vi "LaserMaster.vi"() -> ()   [LabVIEW 2010]
uses:
  <vilib>/Instr/_visa.llb/VISA Configure Serial Port (Instr).vi
  <vilib>/Utility/file.llb/Write To Spreadsheet File (string).vi
panel:
  out "Start time":timestamp
  out "Step":dbl
  out "State next step":string
  in  "stop":bool
  out "Query backup List":string[][](array[string])=[["?L", " 0\r"], ["?K", " 0\r"], ["?F", " 0\r"], ["?FH", " 2\r"], ["?SHUTTER", " 0\r"], ["?UF", " 0\r"], ["?PHLDC", " 1\r"], ["?PZTMC", " 0\r"], ["?PZTXC", " 2.24\r"], ["?PZTYC", " 2.14\r"], ["?PHLDP", " 0\r"], ["?PZTMP", " 0\r"], ["?PZTXP", " 2.58\r"], ["?PXTYP", "  Query Error:?PXTYP\r"], ["?PTRK", "  Query Error:?PTRK\r"], ["?MDLK", " 0\r"], ["?PP", " 0.80\r"], ["?TS", " 0\r"], ["?SM", " 1\r"], ["?HM", " 1\r"], ["?VW", " 850\r"], ["?STPRPOS", " 2096\r"], ["?C", " 0.00\r"], ["?D1C", " 0.08\r"], ["?D2C", " -0.43\r"], ["?BT", " 20.07\r"], ["?D1T", " 24.20\r"], ["?D2T", " 24.20\r"], ["?VT", " 20.72\r"], ["?LBOT", " 148.45\r"], ["?ET", " 39.01\r"], ["?D1ST", " 24.20\r"], ["?D2ST", " 24.20\r"], ["?VST", " 30.00\r"], ["?LBOST", " 148.41\r"], ["?EST", " 39.00\r"], ["?D1TD", " 500.12\r"], ["?D2TD", " 464.53\r"], ["?VD", " 0.00\r"], ["?LBOD", " 5358.08\r"], ["?ED", " 2152.46\r"], ["?D1HST", " 21.35\r"], ["?D2HST", " 21.48\r"], ["?LBOH", " 1\r"], ["?LRS", " 2\r"], ["?D1SS", " 1\r"], ["?D2SS", " 1\r"], ["?VSS", " 0\r"], ["?LBOSS", " 1\r"], ["?ESS", " 1\r"], ["?D1H", "  351.54\r"], ["?D2H", "  351.52\r"], ["?HH", " 37\r"], ["?D1V", " 0.19\r"], ["?D2V", " 0.18\r"], ["?SV", " 8.26,8.26,9.57\r"], ["?MB", "  Query Error:?MB\r"], ["?PI", " 2BC\r"], ["?BV", " 13.24\r"], ["?AMDLK", " 1\r"], ["?PZTS", "  Query Error:?PZTS\r"], ["?TMAX", " 1080\r"], ["?TMIN", " 680\r"], ["?ALIGN", " 0\r"], ["?ALIGNP", " 250\r"], ["?ALIGNW", " 730\r"], ["?LFP", " 0\r"], ["?PZTXCM", " 8.11\r"], ["?PZTXCP", " -10.30\r"], ["?PZTXPM", " 8.11\r"], ["?PZTXPP", " 3.06\r"], ["?PZTYCM", " 8.11\r"], ["?PZTYCP", " -14.28\r"], ["?PZTYPM", " 8.11\r"], ["?PZTYPP", " 11.74\r"], ["?RH", " 0\r"], ["?SN", " 9571\r"], ["?ST", " Standby\r"], ["?GDDCURVE", " 0\r"], ["?GDD", " 0\r"], ["?GDDCURVEN", " ZERO\r"], ["?CURVEN", " OUT OF RANGE\r"], ["?COMP", " 1\r"], ["?HMCOMP", " 1\r"], ["?GDDMAX", " 17333\r"], ["?GDDMIN", "0"]]
  out "Laser Info":i32
  out "Shutter off time":dbl
  out "Quiting":dbl
  out "Backuper state":string
  in  "Tab Control":T1(tab)
  out "Laser Status":bool
  out "Power (mW)":dbl(knob) scale=0.0..5000.0
  out "Walking":bool
  out "Sleeping":bool
  out "ModeLocked":bool
  out "Backing up":bool
  in  "Dither hold":bool
  in  "Shutter":bool
  in  "Wavelength":dbl
  in  "GDD":dbl
  in  "Align":bool
  in  "QUIT":bool
  out "Max":string
  in  "Home motor":bool
  in  "Optimize":bool
  in  "WV Walk":bool
  in  "Auto-Standby\nTime (min)":dbl=120.0
  in  "Sleep":bool
  in  "Backup":bool
  in  "Auto-Backup \nIdle Time (min)":dbl=30.0
  out "Operating Status":string
  out "Tunning Status":i32
  out "Idle Time":dbl format="%.1f"
  out "Laser On Time":dbl format="%#.1f"
  in  "Laser Control":bool
  in  "Refresh":bool
  out "Query List":string[][](array[string])
  out "queue #":i32
  in  "Command Line":string
  out "Laser Response":string
  # "LASER"
  # "LASER fine-tune"
  # "BACKUP"
  # "Timers"
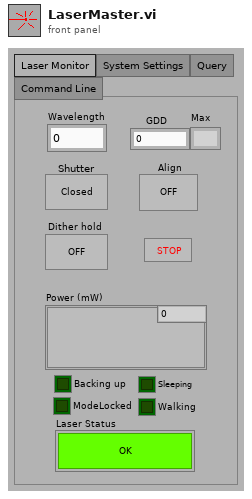
[diagram p1: front panel]
types:
  T1 = enum32{"Laser Monitor", "System Settings", "Query", "Command Line"}
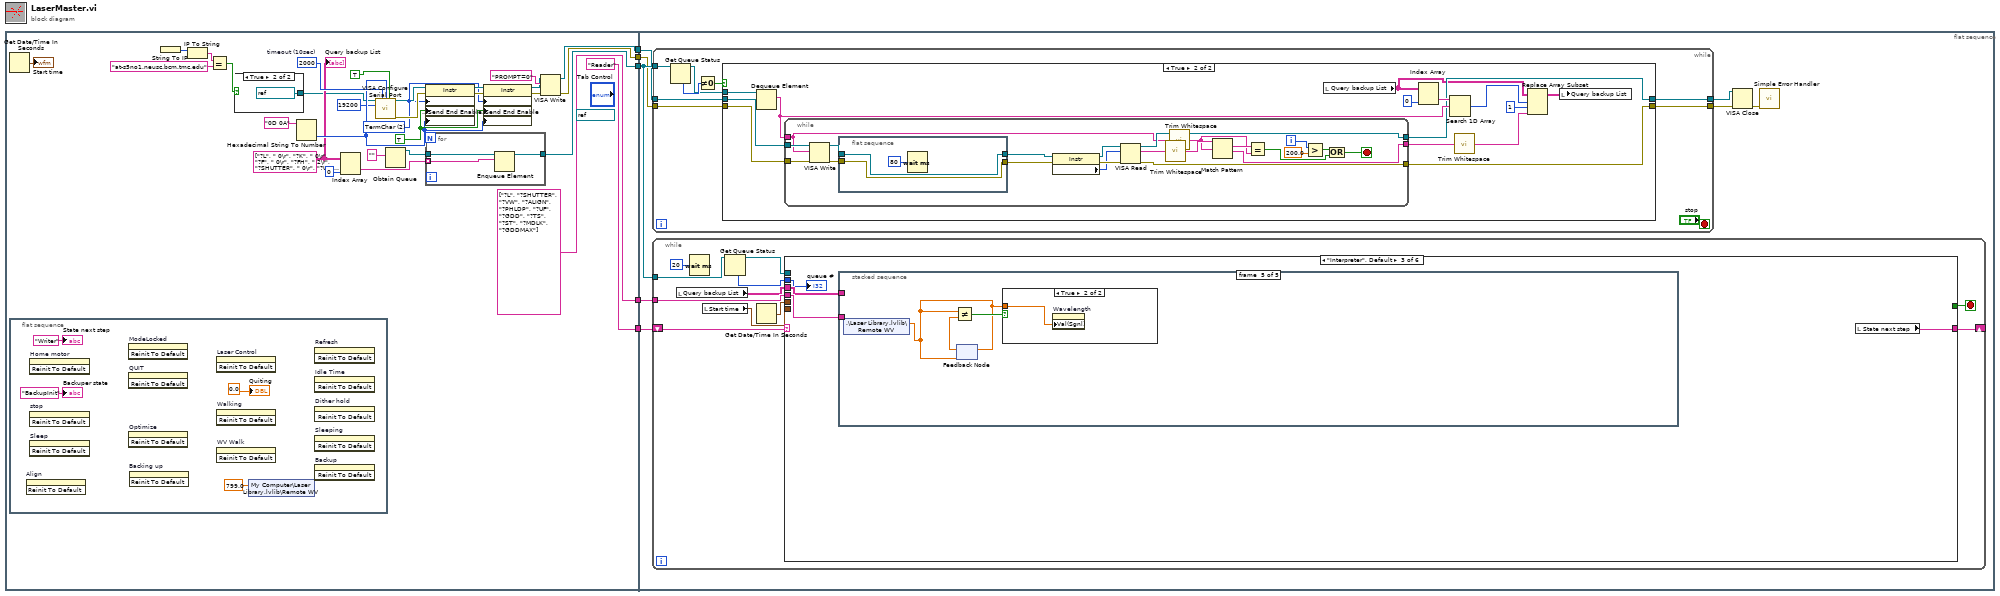
[diagram p0: block diagram]
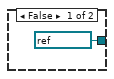
[diagram p2: hidden frame]
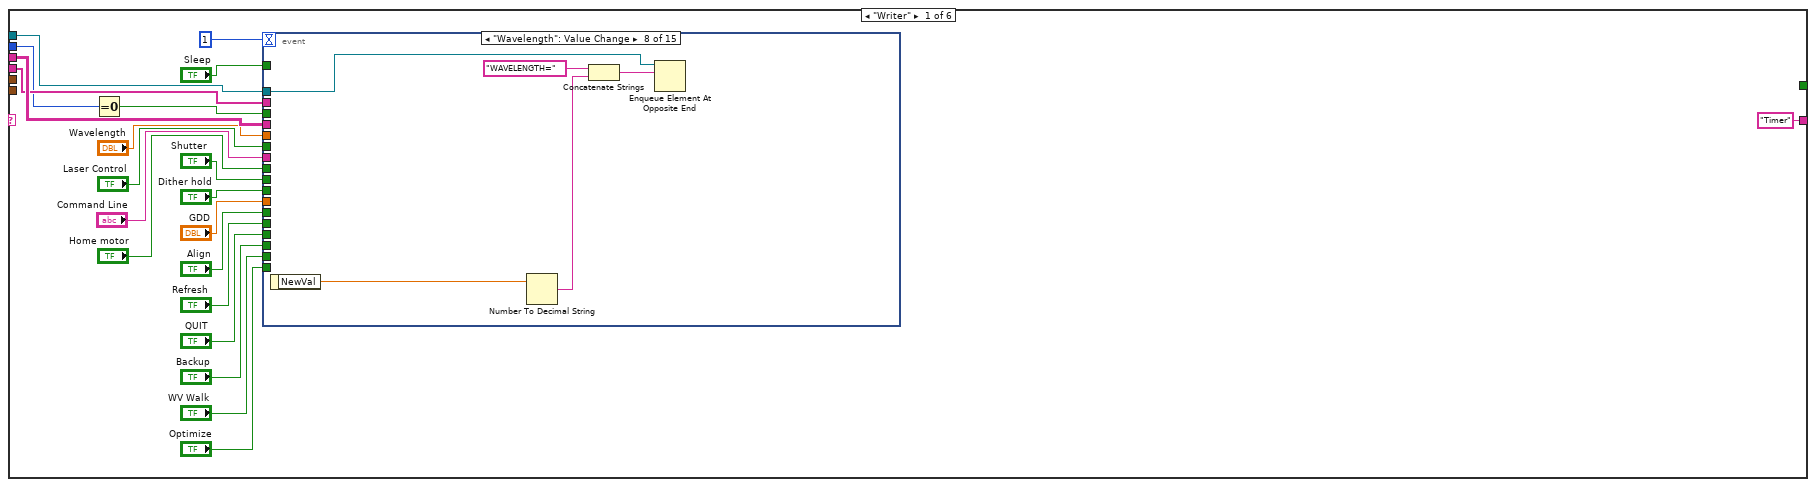
[diagram p4: hidden frame]
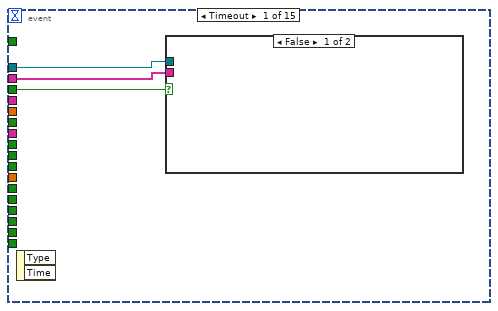
[diagram p5: hidden frame]
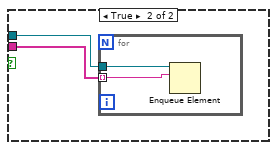
[diagram p6: hidden frame]
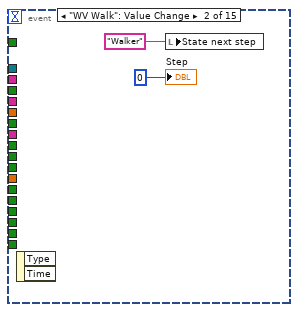
[diagram p7: hidden frame]
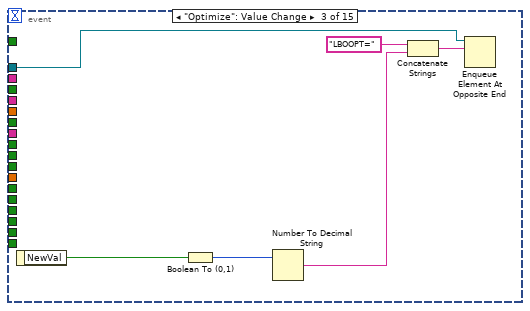
[diagram p8: hidden frame]
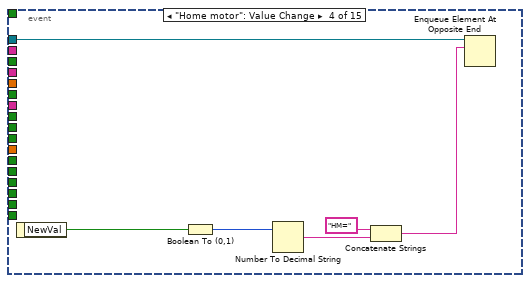
[diagram p9: hidden frame]
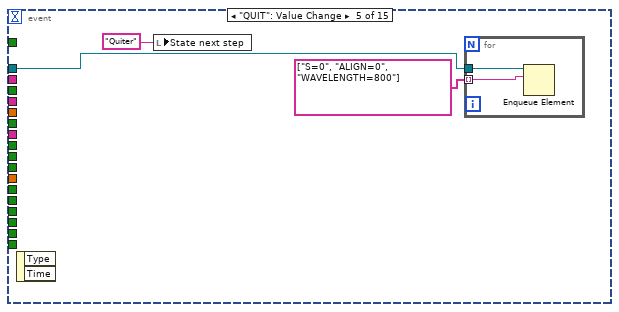
[diagram p10: hidden frame]
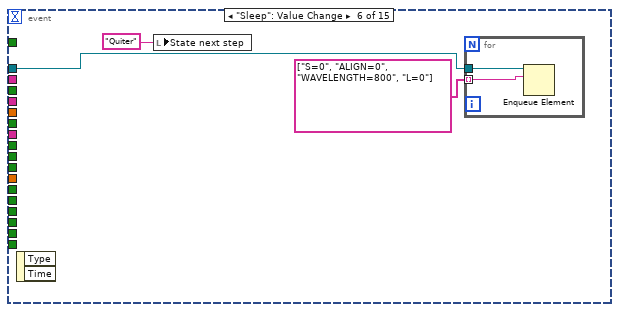
[diagram p11: hidden frame]
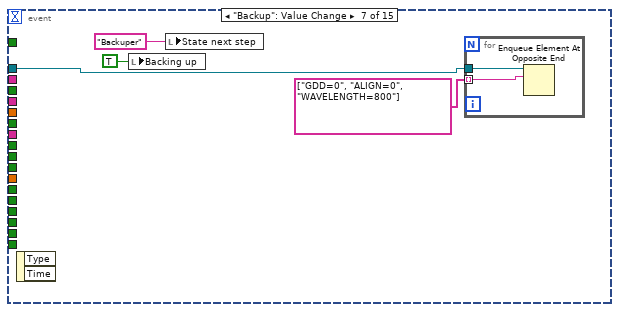
[diagram p12: hidden frame]
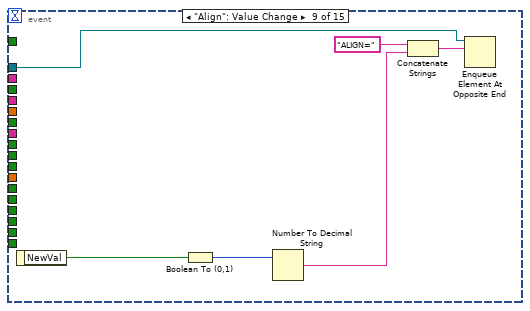
[diagram p13: hidden frame]
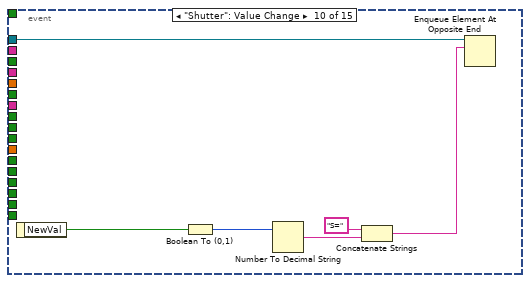
[diagram p14: hidden frame]
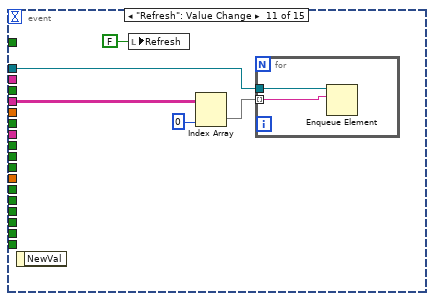
[diagram p15: hidden frame]
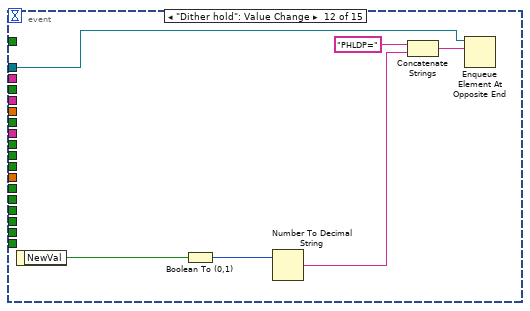
[diagram p16: hidden frame]
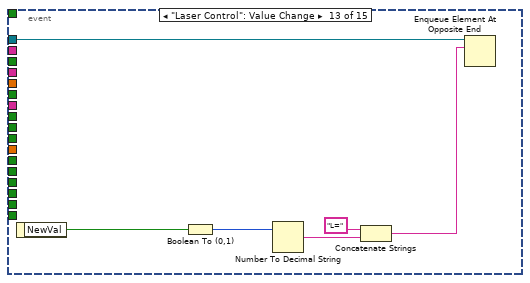
[diagram p17: hidden frame]
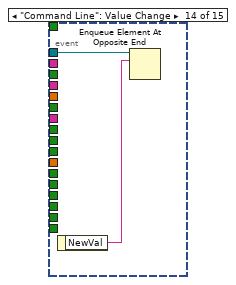
[diagram p18: hidden frame]
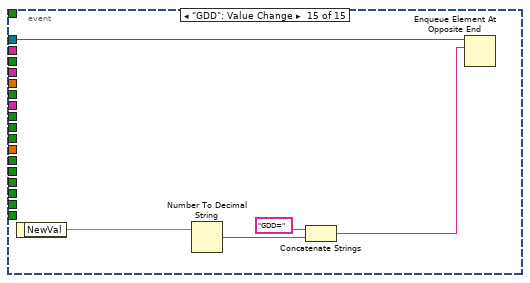
[diagram p19: hidden frame]
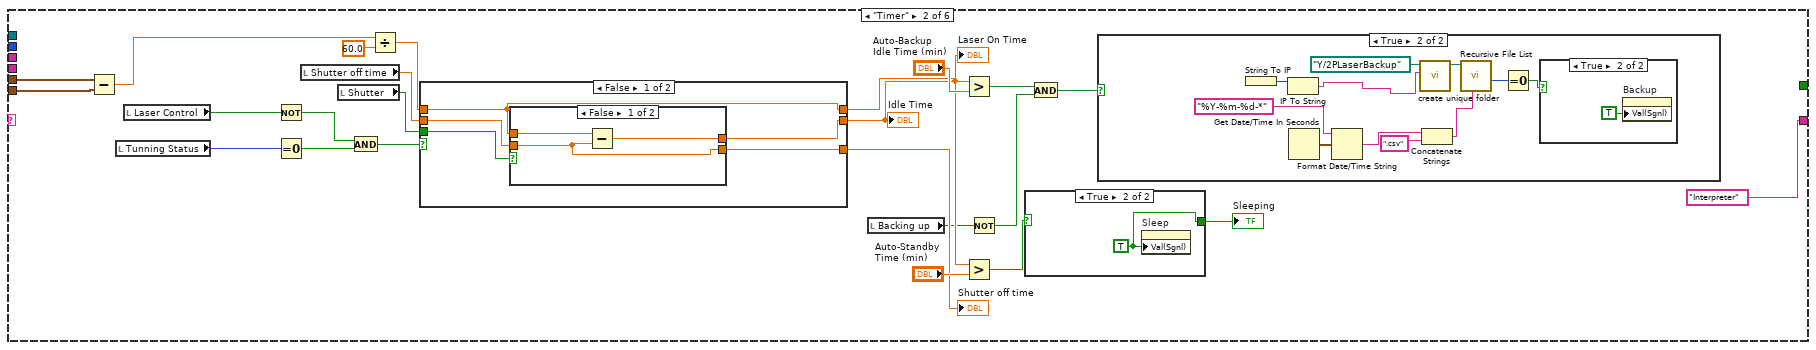
[diagram p20: hidden frame]
diagram:
  n1 = flat-sequence {
    tunnel: [w24] -> w5
    tunnel: [w23] -> w4
    tunnel: [w14] -> w3
    tunnel: [string[] ["?L", "?SHUTTER", "?VW", "?ALIGN", "?PHLDP", "?UF", "?GDD", "?TS", "?ST", "?MDLK", "?GDDMAX"]] -> w2
    tunnel: ["Reader"] -> w1
    tunnel: w5 -> [w48]
    tunnel: w4 -> [w45]
    tunnel: w3 -> [w49]
    tunnel: w2 -> [w51]
    tunnel: w1 -> [w50]
    frame #0 {
      (unwired) refnum<visa-resource-name> "COM1" ("VISA resource name")
      w13 = string[][] [["?L", " 0\r"], ["?K", " 0\r"], ["?F", " 0\r"], ["?FH", " 2\r"], ["?SHUTTER", " 0\r"], ["?UF", " 0\r"], ["?PHLDC", " 1\r"], ["?PZTMC", " 0\r"], ["?PZTXC", " 2.24\r"], ["?PZTYC", " 2.14\r"], ["?PHLDP", " 0\r"], ["?PZTMP", " 0\r"], ["?PZTXP", " 2.58\r"], ["?PXTYP", "  Query Error:?PXTYP\r"], ["?PTRK", "  Query Error:?PTRK\r"], ["?MDLK", " 0\r"], ["?PP", " 0.80\r"], ["?TS", " 0\r"], ["?SM", " 1\r"], ["?HM", " 1\r"], ["?VW", " 850\r"], ["?STPRPOS", " 2096\r"], ["?C", " 0.00\r"], ["?D1C", " 0.08\r"], ["?D2C", " -0.43\r"], ["?BT", " 20.07\r"], ["?D1T", " 24.20\r"], ["?D2T", " 24.20\r"], ["?VT", " 20.72\r"], ["?LBOT", " 148.45\r"], ["?ET", " 39.01\r"], ["?D1ST", " 24.20\r"], ["?D2ST", " 24.20\r"], ["?VST", " 30.00\r"], ["?LBOST", " 148.41\r"], ["?EST", " 39.00\r"], ["?D1TD", " 500.12\r"], ["?D2TD", " 464.53\r"], ["?VD", " 0.00\r"], ["?LBOD", " 5358.08\r"], ["?ED", " 2152.46\r"], ["?D1HST", " 21.35\r"], ["?D2HST", " 21.48\r"], ["?LBOH", " 1\r"], ["?LRS", " 2\r"], ["?D1SS", " 1\r"], ["?D2SS", " 1\r"], ["?VSS", " 0\r"], ["?LBOSS", " 1\r"], ["?ESS", " 1\r"], ["?D1H", "  351.54\r"], ["?D2H", "  351.52\r"], ["?HH", " 37\r"], ["?D1V", " 0.19\r"], ["?D2V", " 0.18\r"], ["?SV", " 8.26,8.26,9.57\r"], ["?MB", "  Query Error:?MB\r"], ["?PI", " 2BC\r"], ["?BV", " 13.24\r"], ["?AMDLK", " 1\r"], ["?PZTS", "  Query Error:?PZTS\r"], ["?TMAX", " 1080\r"], ["?TMIN", " 680\r"], ["?ALIGN", " 0\r"], ["?ALIGNP", " 250\r"], ["?ALIGNW", " 730\r"], ["?LFP", " 0\r"], ["?PZTXCM", " 8.11\r"], ["?PZTXCP", " -10.30\r"], ["?PZTXPM", " 8.11\r"], ["?PZTXPP", " 3.06\r"], ["?PZTYCM", " 8.11\r"], ["?PZTYCP", " -14.28\r"], ["?PZTYPM", " 8.11\r"], ["?PZTYPP", " 11.74\r"], ["?RH", " 0\r"], ["?SN", " 9571\r"], ["?ST", " Standby\r"], ["?GDDCURVE", " 0\r"], ["?GDD", " 0\r"], ["?GDDCURVEN", " ZERO\r"], ["?CURVEN", " OUT OF RANGE\r"], ["?COMP", " 1\r"], ["?HMCOMP", " 1\r"], ["?GDDMAX", " 17333\r"], ["?GDDMIN", "0"]] ("Query backup List")
      w27 = TRUE ("Message Based Settings:Send End Enable")
      w28 = u16 2 items=["None", "LastBit", "TermChar", "Break"] ("Serial Settings:Serial End Mode for Writes")
      w35 = u32 2000  # timeout (10sec)
      n2 = Get Date/Time In Seconds() -> (seconds since 1Jan1904=→"Start time":timestamp)
      n3 = flat-sequence {
        frame #0 {
          n4 = invoke on="Align" class="Bool (strict)" method="Reinit To Default"() -> ()  [unwired: 3 in, 3 out]
          n5 = invoke on="Home motor" class="Bool" method="Reinit To Default"() -> ()  [unwired: 3 in, 3 out]
          n6 = invoke on="stop" class="Bool (strict)" method="Reinit To Default"() -> ()  [unwired: 3 in, 3 out]
          n7 = invoke on="Sleep" class="Bool (strict)" method="Reinit To Default"() -> ()  [unwired: 3 in, 3 out]
          n8 = invoke on="ModeLocked" class="Bool (strict)" method="Reinit To Default"() -> ()  [unwired: 3 in, 3 out]
          n9 = invoke on="QUIT" class="Bool (strict)" method="Reinit To Default"() -> ()  [unwired: 3 in, 3 out]
          n10 = invoke on="Optimize" class="Bool" method="Reinit To Default"() -> ()  [unwired: 3 in, 3 out]
          n11 = invoke on="Backing up" class="Bool (strict)" method="Reinit To Default"() -> ()  [unwired: 3 in, 3 out]
          n12 = invoke on="Laser Control" class="Bool (strict)" method="Reinit To Default"() -> ()  [unwired: 3 in, 3 out]
          n13 = invoke on="Walking" class="Bool (strict)" method="Reinit To Default"() -> ()  [unwired: 3 in, 3 out]
          n14 = invoke on="WV Walk" class="Bool (strict)" method="Reinit To Default"() -> ()  [unwired: 3 in, 3 out]
          n15 = shared-variable "My Computer\\Laser Library.lvlib\\Remote WV"(799.0 ("Remote WV")) -> ()  [unwired: 1 in, 1 out]
          n16 = invoke on="Refresh" class="Bool (strict)" method="Reinit To Default"() -> ()  [unwired: 3 in, 3 out]
          n17 = invoke on="Idle Time" class="DigNum (strict)" method="Reinit To Default"() -> ()  [unwired: 3 in, 3 out]
          n18 = invoke on="Dither hold" class="Bool (strict)" method="Reinit To Default"() -> ()  [unwired: 3 in, 3 out]
          n19 = invoke on="Sleeping" class="Bool (strict)" method="Reinit To Default"() -> ()  [unwired: 3 in, 3 out]
          n20 = invoke on="Backup" class="Bool (strict)" method="Reinit To Default"() -> ()  [unwired: 3 in, 3 out]
          "Backuper state" <- "BackupInit"
          "Quiting" <- 0.0 ("Quiting")
          "State next step" <- "Writer"
        }
      }
      n21 = String To IP() -> (0:w10:u32)  [unwired: 1 in]
      n22 = IP To String(2:w10) -> (0:w9:string)  [unwired: 1 in]
      n23 = Equal?(x=w9, y="at-s5no1.neusc.bcm.tmc.edu") -> (x = y?=w6:bool)
      n24 = case shown="True" w6 {
        tunnel: [refnum<visa-resource-name> "COM1" ("VISA resource name") refnum<visa-resource-name> "COM5" ("VISA resource name")] -> w7
        frame False {
        }
        frame True {
        }
      }
      n25 = Hexadecimal String To Number(string="0D 0A") -> (number=w26:u32)  [unwired: 2 in, 1 out]
      n26 = Index Array(array=w13, index (col)=0 ("disabled index (col)")) -> (element=w16:string[])  [unwired: 1 in]
      n27 = call-poly "VISA Configure Serial Port"("VISA resource name"=w7, "timeout (10sec)"=w35, "termination char\n(0xA = '\\n' = LF)"=w26, "Enable Termination\nChar (T)"=TRUE ("Enable Termination\nChar (T)"), "baud rate (9600)"=u32 19200) -> ("VISA resource name out"=w32:refnum<visa-resource-name>, "error out"=w31:errorcluster)  [unwired: 5 in, 4 out]
      n28 = Obtain Queue(element data type="") -> (queue out=w18:refnum<queue>)  [unwired: 4 in, 2 out]
      n29 = property class="Instr"(reference=w32, error in=w31, "Serial Settings:End Mode for Writes"=w28, "Message Based Settings:Send End Enable"=w27, "Message Based Settings:Termination Character"=w26) -> (reference out=w30:refnum<visa-resource-name>, error out=w29:errorcluster)
      n30 = for {
        tunnel: w18 -> [w44]
        tunnel: w16 -> [w43] mode=indexing
        tunnel: [w42] -> w14
        n31 = Enqueue Element(queue=w44, element=w43) -> (queue out=w42:refnum<queue>)  [unwired: 2 in, 2 out]
      }
      n32 = property class="Instr"(reference=w30, error in=w29, "Serial Settings:End Mode for Writes"=w28, "Message Based Settings:Send End Enable"=w27, "Message Based Settings:Termination Character"=w26) -> (reference out=w21:refnum<visa-resource-name>, error out=w20:errorcluster)
      n33 = VISA Write(VISA resource name=w21, write buffer="PROMPT=0", error in (no error)=w20) -> (VISA resource name out=w24:refnum<visa-resource-name>, error out=w23:errorcluster)  [unwired: 1 out]
      "Query backup List" <- w13
    }
    frame #1 {
      n34 = while {
        tunnel: w49 -> [w56]
        tunnel: w48 -> [w61]
        tunnel: [w60] -> w47
        tunnel: [w59] -> w46
        tunnel: w45 -> [w58]
        stop <- "stop" stop-if-true
        n35 = Get Queue Status(queue=w56) -> (queue out=w53:refnum<queue>, # elements in queue=w55:i32)  [unwired: 2 in, 6 out]
        n36 = Not Equal To 0?(x=w55) -> (x != 0?=w54:bool)
        n37 = case shown="True" w54 {
          tunnel: w53 -> [_ w70]
          tunnel: w61 -> [w63 w69]
          tunnel: [w63 w68] -> w60
          tunnel: [w62 w67] -> w59
          tunnel: w58 -> [w62 w66]
          frame False {
          }
          frame True {
            n38 = Dequeue Element(queue=w70) -> (element=w72:string)  [unwired: 2 in, 3 out]
            n39 = while {
              tunnel: w69 -> [w99]
              tunnel: w66 -> [w98]
              tunnel: [w97] -> w68
              tunnel: [w96] -> w67
              tunnel: w72 -> [w84]
              tunnel: [w92] -> w73
              i -> [w82]
              stop <- w79 stop-if-true
              n40 = VISA Write(VISA resource name=w99, write buffer=w84, error in (no error)=w98) -> (VISA resource name out=w90:refnum<visa-resource-name>, error out=w87:errorcluster)  [unwired: 1 out]
              n41 = flat-sequence {
                tunnel: [w102] -> w89
                tunnel: w90 -> [w102]
                tunnel: w87 -> [w101]
                tunnel: [w101] -> w88
                frame #0 {
                  n42 = Wait (ms)(milliseconds to wait=u32 80) -> ()  [unwired: 1 out]
                }
              }
              n43 = property class="Instr"(reference=w89, error in=w88) -> (reference out=w95:refnum<visa-resource-name>, error out=w94:errorcluster, "Serial Settings:Number of Bytes at Serial Port"=w93:u32)
              n44 = VISA Read(VISA resource name=w95, byte count=w93, error in (no error)=w94) -> (VISA resource name out=w97:refnum<visa-resource-name>, read buffer=w86:string, error out=w96:errorcluster)  [unwired: 1 out]
              n45 = call <vilib>:"Trim Whitespace.vi"("string"=w86) -> ("trimmed string"=w85:string)  [unwired: 1 in]
              n46 = call <vilib>:"Trim Whitespace.vi"("string"=w84) -> ("trimmed string"=w78:string)  [unwired: 1 in]
              n47 = Match Pattern(string=w85, regular expression=w78) -> (match substring=w91:string, after substring=w92:string)  [unwired: 1 in, 2 out]
              n48 = Equal?(x=w91, y=w78) -> (x = y?=w80:bool)
              n49 = Greater?(x=w82, y=200.0) -> (0:w81:bool)
              n50 = Compound Arithmetic op=OR(w81, w80) -> (w79:bool)
            }
            n51 = local read "Query backup List"() -> (w65:string[][])
            n52 = Index Array(array=w65, index (col)=0 ("index (row)")) -> (element=w76:string[])  [unwired: 1 in]
            n53 = Search 1D Array(1D array=w76, element=w72) -> (index of element=w74:i32)  [unwired: 1 in]
            n54 = call <vilib>:"Trim Whitespace.vi"("string"=w73) -> ("trimmed string"=w71:string)  [unwired: 1 in]
            n55 = Replace Array Subset(array=w65, new element=w71, index (row)=w74, index (col)=1 ("disabled index (col)")) -> (w64:string[][])
            n56 = local write "Query backup List"(w64) -> ()
          }
        }
      }
      n57 = while {
        tunnel: w49 -> [w110]
        tunnel: w51 -> [w111]
        shift-right: [w112] -> _
        shift-left: w50 -> [w113]
        stop <- w107 stop-if-true
        n58 = local read "Query backup List"() -> (w109:string[][])
        n59 = Wait (ms)(milliseconds to wait=u32 20) -> ()  [unwired: 1 out]
        n60 = local read "Start time"() -> (w103:timestamp)
        n61 = Get Queue Status(queue=w110) -> (queue out=w106:refnum<queue>, # elements in queue=w105:i32)  [unwired: 2 in, 6 out]
        n62 = Get Date/Time In Seconds() -> (seconds since 1Jan1904=w104:timestamp)
        n63 = case shown="\"Interpreter\", Default" w113 {
          tunnel: w106 -> [w134 _ _ _ _ _]
          tunnel: w109 -> [w133 _ w267 _ w400 _]
          tunnel: w111 -> [w132 _ w268 _ _ _]
          tunnel: ["Timer" "Interpreter" w266 "Writer" "Writer" w425] -> w112
          tunnel: w105 -> [w131 _ w265 _ _ w427]
          tunnel: [_ _ _ _ _ w424] -> w107
          tunnel: w104 -> [_ w218 _ _ _ _]
          tunnel: w103 -> [_ w216 _ _ _ _]
          frame "Writer" {
            n64 = Equal To 0?(x=w131) -> (x = 0?=w119:bool)
            n65 = event shown="[7] \"Wavelength\": Value Change" {
              selector: _ -> [_ _ _ _ _ _ _ _ _ _ _ _ _ _ _]
              dyn-events: _ -> [_ _ _ _ _ _ _ _ _ _ _ _ _ _ _]
              timeout: 1 -> [_ _ _ _ _ _ _ _ _ _ _ _ _ _ _]
              tunnel: w134 -> [w137 _ w144 w151 w157 w161 w168 w173 w178 w184 w190 w197 w202 w209 w211]
              tunnel: "Shutter" -> [_ _ _ _ _ _ _ _ _ _ _ _ _ _ _]
              tunnel: "Dither hold" -> [_ _ _ _ _ _ _ _ _ _ _ _ _ _ _]
              tunnel: "GDD" -> [_ _ _ _ _ _ _ _ _ _ _ _ _ _ _]
              tunnel: "Align" -> [_ _ _ _ _ _ _ _ _ _ _ _ _ _ _]
              tunnel: "Wavelength" -> [_ _ _ _ _ _ _ _ _ _ _ _ _ _ _]
              tunnel: "Laser Control" -> [_ _ _ _ _ _ _ _ _ _ _ _ _ _ _]
              tunnel: "Command Line" -> [_ _ _ _ _ _ _ _ _ _ _ _ _ _ _]
              tunnel: w133 -> [_ _ _ _ _ _ _ _ _ _ w189 _ _ _ _]
              tunnel: "Refresh" -> [_ _ _ _ _ _ _ _ _ _ _ _ _ _ _]
              tunnel: w132 -> [w136 _ _ _ _ _ _ _ _ _ _ _ _ _ _]
              tunnel: "QUIT" -> [_ _ _ _ _ _ _ _ _ _ _ _ _ _ _]
              tunnel: "Backup" -> [_ _ _ _ _ _ _ _ _ _ _ _ _ _ _]
              tunnel: w119 -> [w135 _ _ _ _ _ _ _ _ _ _ _ _ _ _]
              tunnel: "WV Walk" -> [_ _ _ _ _ _ _ _ _ _ _ _ _ _ _]
              tunnel: "Optimize" -> [_ _ _ _ _ _ _ _ _ _ _ _ _ _ _]
              tunnel: "Home motor" -> [_ _ _ _ _ _ _ _ _ _ _ _ _ _ _]
              tunnel: "Sleep" -> [_ _ _ _ _ _ _ _ _ _ _ _ _ _ _]
              event Timeout {
                n66 = event-data() -> ()  [unwired: 1 in, 2 out]
                n67 = case shown="False" w135 {
                  tunnel: w137 -> [_ w139]
                  tunnel: w136 -> [_ w138]
                  frame False {
                  }
                  frame True {
                    n68 = for {
                      tunnel: w139 -> [w141]
                      tunnel: w138 -> [w140] mode=indexing
                      n69 = Enqueue Element(queue=w141, element=w140) -> ()  [unwired: 2 in, 3 out]
                    }
                  }
                }
              }
              event "WV Walk": Value Change {
                n70 = event-data() -> ()  [unwired: 1 in, 2 out]
                n71 = local write "State next step"("Walker") -> ()
                "Step" <- 0
              }
              event "Optimize": Value Change {
                n72 = event-data() -> ("NewVal"=w145:bool)  [unwired: 1 in]
                n73 = Boolean To (0,1)(Boolean=w145) -> (0, 1=w148:i16)
                n74 = Number To Decimal String(number=w148) -> (decimal integer string=w149:string)  [unwired: 1 in]
                n75 = Concatenate Strings("LBOOPT=", w149) -> (w146:string)
                n76 = Enqueue Element At Opposite End(queue=w144, element=w146) -> ()  [unwired: 2 in, 3 out]
              }
              event "Home motor": Value Change {
                n77 = event-data() -> ("NewVal"=w150:bool)  [unwired: 1 in]
                n78 = Boolean To (0,1)(Boolean=w150) -> (0, 1=w154:i16)
                n79 = Number To Decimal String(number=w154) -> (decimal integer string=w155:string)  [unwired: 1 in]
                n80 = Concatenate Strings("HM=", w155) -> (w152:string)
                n81 = Enqueue Element At Opposite End(queue=w151, element=w152) -> ()  [unwired: 2 in, 3 out]
              }
              event "QUIT": Value Change {
                n82 = event-data() -> ()  [unwired: 1 in, 2 out]
                n83 = local write "State next step"("Quiter") -> ()
                n84 = for {
                  tunnel: w157 -> [w160]
                  tunnel: string[] ["S=0", "ALIGN=0", "WAVELENGTH=800"] -> [w159] mode=indexing
                  n85 = Enqueue Element(queue=w160, element=w159) -> ()  [unwired: 2 in, 3 out]
                }
              }
              event "Sleep": Value Change {
                n86 = event-data() -> ()  [unwired: 1 in, 2 out]
                n87 = local write "State next step"("Quiter") -> ()
                n88 = for {
                  tunnel: w161 -> [w165]
                  tunnel: string[] ["S=0", "ALIGN=0", "WAVELENGTH=800", "L=0"] -> [w164] mode=indexing
                  n89 = Enqueue Element(queue=w165, element=w164) -> ()  [unwired: 2 in, 3 out]
                }
              }
              event "Backup": Value Change {
                n90 = event-data() -> ()  [unwired: 1 in, 2 out]
                n91 = local write "Backing up"(TRUE ("Backing up ...")) -> ()
                n92 = local write "State next step"("Backuper") -> ()
                n93 = for {
                  tunnel: string[] ["GDD=0", "ALIGN=0", "WAVELENGTH=800"] -> [w171] mode=indexing
                  tunnel: w168 -> [w170]
                  n94 = Enqueue Element At Opposite End(queue=w170, element=w171) -> ()  [unwired: 2 in, 3 out]
                }
              }
              event "Wavelength": Value Change {
                n95 = event-data() -> ("NewVal"=w172:dbl)  [unwired: 1 in]
                n96 = Number To Decimal String(number=w172) -> (decimal integer string=w175:string)  [unwired: 1 in]
                n97 = Concatenate Strings("WAVELENGTH=", w175) -> (w176:string)
                n98 = Enqueue Element At Opposite End(queue=w173, element=w176) -> ()  [unwired: 2 in, 3 out]
              }
              event "Align": Value Change {
                n99 = event-data() -> ("NewVal"=w177:bool)  [unwired: 1 in]
                n100 = Boolean To (0,1)(Boolean=w177) -> (0, 1=w181:i16)
                n101 = Number To Decimal String(number=w181) -> (decimal integer string=w182:string)  [unwired: 1 in]
                n102 = Concatenate Strings("ALIGN=", w182) -> (w179:string)
                n103 = Enqueue Element At Opposite End(queue=w178, element=w179) -> ()  [unwired: 2 in, 3 out]
              }
              event "Shutter": Value Change {
                n104 = event-data() -> ("NewVal"=w183:bool)  [unwired: 1 in]
                n105 = Boolean To (0,1)(Boolean=w183) -> (0, 1=w187:i16)
                n106 = Number To Decimal String(number=w187) -> (decimal integer string=w188:string)  [unwired: 1 in]
                n107 = Concatenate Strings("S=", w188) -> (w185:string)
                n108 = Enqueue Element At Opposite End(queue=w184, element=w185) -> ()  [unwired: 2 in, 3 out]
              }
              event "Refresh": Value Change {
                n109 = event-data() -> ()  [unwired: 1 in, 1 out]
                n110 = local write "Refresh"(FALSE ("Backup")) -> ()
                n111 = Index Array(array=w189, index (col)=0 ("disabled index (col)")) -> (element=w192:string[])  [unwired: 1 in]
                n112 = for {
                  tunnel: w190 -> [w195]
                  tunnel: w192 -> [w194] mode=indexing
                  n113 = Enqueue Element(queue=w195, element=w194) -> ()  [unwired: 2 in, 3 out]
                }
              }
              event "Dither hold": Value Change {
                n114 = event-data() -> ("NewVal"=w196:bool)  [unwired: 1 in]
                n115 = Boolean To (0,1)(Boolean=w196) -> (0, 1=w200:i16)
                n116 = Number To Decimal String(number=w200) -> (decimal integer string=w201:string)  [unwired: 1 in]
                n117 = Concatenate Strings("PHLDP=", w201) -> (w198:string)
                n118 = Enqueue Element At Opposite End(queue=w197, element=w198) -> ()  [unwired: 2 in, 3 out]
              }
              event "Laser Control": Value Change {
                n119 = event-data() -> ("NewVal"=w203:bool)  [unwired: 1 in]
                n120 = Boolean To (0,1)(Boolean=w203) -> (0, 1=w206:i16)
                n121 = Number To Decimal String(number=w206) -> (decimal integer string=w207:string)  [unwired: 1 in]
                n122 = Concatenate Strings("L=", w207) -> (w204:string)
                n123 = Enqueue Element At Opposite End(queue=w202, element=w204) -> ()  [unwired: 2 in, 3 out]
              }
              event "Command Line": Value Change {
                n124 = event-data() -> ("NewVal"=w208:string)  [unwired: 1 in]
                n125 = Enqueue Element At Opposite End(queue=w209, element=w208) -> ()  [unwired: 2 in, 3 out]
              }
              event "GDD": Value Change {
                n126 = event-data() -> ("NewVal"=w210:dbl)  [unwired: 1 in]
                n127 = Number To Decimal String(number=w210) -> (decimal integer string=w213:string)  [unwired: 1 in]
                n128 = Concatenate Strings("GDD=", w213) -> (w214:string)
                n129 = Enqueue Element At Opposite End(queue=w211, element=w214) -> ()  [unwired: 2 in, 3 out]
              }
            }
          }
          frame "Timer" {
            n130 = Subtract(x=w218, y=w216) -> (x-y=w220:dbl)
            n131 = local read "Tunning Status"() -> (w237:i32)
            n132 = local read "Laser Control"() -> (w236:bool)
            n133 = Not(x=w236) -> (.not. x?=w232:bool)
            n134 = Equal To 0?(x=w237) -> (x = 0?=w231:bool)
            n135 = local read "Shutter off time"() -> (w227:dbl)
            n136 = local read "Shutter"() -> (w228:bool)
            n137 = And(x=w232, y=w231) -> (x .and. y?=w233:bool)
            n138 = Divide(x=w220, y=60.0 ("x")) -> (x/y=w217:dbl)
            n139 = case shown="False" w233 {
              tunnel: [w239 w250] -> w230
              tunnel: [w243 w250] -> w229
              tunnel: w228 -> [w242 _]
              tunnel: w227 -> [w241 _]
              tunnel: [w240 w250] -> w226
              tunnel: w217 -> [w239 _]
              frame False {
                n140 = case shown="False" w242 {
                  tunnel: [w246 0] -> w243
                  tunnel: w239 -> [w245 w247]
                  tunnel: w241 -> [w244 _]
                  tunnel: [w244 w247] -> w240
                  frame False {
                    n141 = Subtract(x=w245, y=w244) -> (x-y=w246:dbl)
                  }
                  frame True {
                  }
                }
              }
              frame True {
                w250 = 0
                n142 = Get Date/Time In Seconds() -> (seconds since 1Jan1904=w249:timestamp)
                n143 = local write "Start time"(w249) -> ()
              }
            }
            "Laser On Time" <- w230
            "Idle Time" <- w229
            "Shutter off time" <- w226
            n144 = local read "Backing up"() -> (w221:bool)
            n145 = Greater?(x=w229, y="Auto-Backup \nIdle Time (min)") -> (0:w224:bool)
            n146 = Greater?(x=w229, y="Auto-Standby\nTime (min)") -> (0:w215:bool)
            n147 = Not(x=w221) -> (.not. x?=w223:bool)
            n148 = case shown="True" w215 {
              tunnel: [FALSE ("Sleeping") w252] -> w225
              frame False {
              }
              frame True {
                w252 = TRUE
                n149 = property on="Sleep" class="Bool (strict)"("Val(Sgnl)"=w252) -> ()  [unwired: 2 in, 2 out]
              }
            }
            "Sleeping" <- w225
            n150 = And(x=w224, y=w223) -> (x .and. y?=w222:bool)
            n151 = case shown="True" w222 {
              frame False {
              }
              frame True {
                n152 = String To IP() -> (0:w256:u32)  [unwired: 1 in]
                n153 = IP To String(2:w256) -> (0:w253:string)  [unwired: 1 in]
                n154 = Get Date/Time In Seconds() -> (seconds since 1Jan1904=w259:timestamp)
                n155 = Format Date/Time String(time format string (%c)="%Y-%m-%d-*", seconds (now)=w259) -> (date/time string=w255:string)  [unwired: 1 in]
                n156 = call "create unique folder.vi"("string"=w253, "path 2"=path "Y:/2PLaserBackup") -> ("path"=w262:path)  [unwired: 9 in]
                n157 = Concatenate Strings(w255, ".csv" ("string")) -> (w261:string)
                n158 = call <vilib>:"Recursive File List.vi"("pattern"=w261, "Folder Path"=w262) -> ("Number of Files"=w263:i32)  [unwired: 5 in, 4 out]
                n159 = Equal To 0?(x=w263) -> (x = 0?=w254:bool)
                n160 = case shown="True" w254 {
                  frame False {
                  }
                  frame True {
                    n161 = property on="Backup" class="Bool (strict)"("Val(Sgnl)"=TRUE) -> ()  [unwired: 2 in, 2 out]
                  }
                }
              }
            }
          }
          frame "Interpreter", Default {
            n162 = stacked-sequence {
              tunnel: w268 -> [_ w277 _ _ _]
              tunnel: w267 -> [w269 w276 _ w349 _]
              frame #0 {
                n163 = Index Array(array=w269, index (col)=0 ("disabled index (col)")) -> (element=w274:string[])  [unwired: 1 in]
                n164 = local read "Command Line"() -> (w273:string)
                n165 = Search 1D Array(1D array=w274, element=w273) -> (index of element=w272:i32)  [unwired: 1 in]
                n166 = Index Array(array=w269, index (row)=w272, index (col)=1 ("disabled index (col)")) -> (element=→"Laser Response":string)
              }
              frame #1 {
                n167 = for {
                  tunnel: w277 -> [w279] mode=indexing
                  tunnel: w276 -> [w280]
                  n168 = Index Array(array=w280, index (col)=0 ("disabled index (col)")) -> (element=w283:string[])  [unwired: 1 in]
                  n169 = Search 1D Array(1D array=w283, element=w279) -> (index of element=w281:i32)  [unwired: 1 in]
                  n170 = Index Array(array=w280, index (row)=w281, index (col)=1 ("disabled index (col)")) -> (element=w278:string)
                  n171 = case shown="\"?GDD\"" w279 {
                    tunnel: w278 -> [_ w285 w287 w295 w296 w303 w310 w313 w321 w323 w325 w327]
                    frame "False", Default {
                    }
                    frame "?L" {
                      n172 = Decimal String To Number(string=w285) -> (number=→"Laser Info":i32)  [unwired: 2 in, 1 out]
                    }
                    frame "?SHUTTER" {
                      n173 = Decimal String To Number(string=w287) -> (number=w288:i32)  [unwired: 2 in, 1 out]
                      n174 = local read "Shutter"() -> (w291:bool)
                      n175 = Not Equal To 0?(x=w288) -> (x != 0?=w290:bool)
                      n176 = And(x=w290, y=w291) -> (x .and. y?=w289:bool)
                      n177 = case shown="False" w289 {
                        frame False {
                          n178 = property on="Shutter" class="Bool (strict)"("Colors [4]"=cluster{u32, u32}[] [{12369084, 12369084}, {12369084, 12369084}]) -> ()  [unwired: 2 in, 2 out]
                        }
                        frame True {
                          n179 = property on="Shutter" class="Bool (strict)"("Colors [4]"=cluster{u32, u32}[] [{12369084, 12369084}, {6618880, 6618880}]) -> ()  [unwired: 2 in, 2 out]
                        }
                      }
                    }
                    frame "?VW" {
                      n180 = Decimal String To Number(string=w295) -> (number=w294:i32)  [unwired: 2 in, 1 out]
                      n181 = property on="Wavelength" class="DigNum (strict)"("Value"=w294) -> ()  [unwired: 2 in, 2 out]
                      n182 = shared-variable ".\\Laser Library.lvlib\\WV"(w294) -> ()  [unwired: 1 in, 1 out]
                    }
                    frame "?ALIGN" {
                      n183 = Decimal String To Number(string=w296) -> (number=w297:i32)  [unwired: 2 in, 1 out]
                      n184 = Not Equal To 0?(x=w297) -> (x != 0?=w300:bool)
                      n185 = local read "Align"() -> (w299:bool)
                      n186 = And(x=w300, y=w299) -> (x .and. y?=w298:bool)
                      n187 = case shown="False" w298 {
                        frame False {
                          n188 = property on="Align" class="Bool (strict)"("Colors [4]"=cluster{u32, u32}[] [{12369084, 12369084}, {12369084, 12369084}]) -> ()  [unwired: 2 in, 2 out]
                        }
                        frame True {
                          n189 = property on="Align" class="Bool (strict)"("Colors [4]"=cluster{u32, u32}[] [{12369084, 12369084}, {6618880, 6618880}]) -> ()  [unwired: 2 in, 2 out]
                        }
                      }
                    }
                    frame "?PHLDP" {
                      n190 = Decimal String To Number(string=w303) -> (number=w304:i32)  [unwired: 2 in, 1 out]
                      n191 = Not Equal To 0?(x=w304) -> (x != 0?=w307:bool)
                      n192 = local read "Dither hold"() -> (w305:bool)
                      n193 = And(x=w307, y=w305) -> (x .and. y?=w306:bool)
                      n194 = case shown="False" w306 {
                        frame False {
                          n195 = property on="Dither hold" class="Bool (strict)"("Colors [4]"=cluster{u32, u32}[] [{12369084, 12369084}, {12369084, 12369084}]) -> ()  [unwired: 2 in, 2 out]
                        }
                        frame True {
                          n196 = property on="Dither hold" class="Bool (strict)"("Colors [4]"=cluster{u32, u32}[] [{12369084, 12369084}, {6618880, 6618880}]) -> ()  [unwired: 2 in, 2 out]
                        }
                      }
                    }
                    frame "?UF" {
                      n197 = Decimal String To Number(string=w310) -> (number=→"Power (mW)":i32)  [unwired: 2 in, 1 out]
                    }
                    frame "?GDD" {
                      n198 = Decimal String To Number(string=w313) -> (number=w312:i32)  [unwired: 2 in, 1 out]
                      n199 = property on="GDD" class="DigNum (strict)"("Value"=w312) -> ()  [unwired: 2 in, 2 out]
                      n200 = shared-variable "My Computer\\Laser Library.lvlib\\GDD"(w312) -> ()  [unwired: 1 in, 1 out]
                    }
                    frame "?GDDMAX" {
                      n201 = Decimal String To Number(string=w321) -> (number=w319:i32)  [unwired: 2 in, 1 out]
                      n202 = Divide(x=w319, y=1000.0) -> (x/y=w315:dbl)
                      n203 = Round To Nearest(number=w315) -> (nearest integer value=w314:dbl)
                      n204 = Number To Decimal String(number=w314) -> (decimal integer string=w318:string)  [unwired: 1 in]
                      n205 = Concatenate Strings(w318, "k" ("string")) -> (→"Max":string)
                    }
                    frame "?TS" {
                      n206 = Decimal String To Number(string=w323) -> (number=→"Tunning Status":i32)  [unwired: 2 in, 1 out]
                    }
                    frame "?MDLK" {
                      n207 = Decimal String To Number(string=w325) -> (number=w326:i32)  [unwired: 2 in, 1 out]
                      n208 = Not Equal To 0?(x=w326) -> (x != 0?=→"ModeLocked":bool)
                    }
                    frame "?ST" {
                      n209 = Initialize Array(w327, 4 ("dimension size")) -> (w329:string[])
                      n210 = property on="Laser Status" class="Bool (strict)"("Strings [4]"=w329) -> ()  [unwired: 2 in, 2 out]
                      "Operating Status" <- w327
                    }
                  }
                }
              }
              frame #2 {
                n211 = local read "Tunning Status"() -> (w330:i32)
                n212 = local read "Laser Info"() -> (w334:i32)
                n213 = Equal To 0?(x=w330) -> (x = 0?=w331:bool)
                n214 = Equal?(x=0, y=w334) -> (x = y?=w332:bool)
                n215 = And(x=w331, y=w332) -> (x .and. y?=w333:bool)
                n216 = Equal?(x=w334, y=2.0) -> (x = y?=w337:bool)
                n217 = case shown="False" w337 {
                  tunnel: w333 -> [w338 _]
                  frame False {
                    n218 = case shown="True" w338 {
                      frame False {
                        w340 = TRUE ("Laser Status")
                        n219 = local read "Operating Status"() -> (w339:string)
                        n220 = local write "Laser Control"(w340) -> ()
                        n221 = local write "Laser Status"(w340) -> ()
                        n222 = Equal?(x=w339, y="OK") -> (x = y?=w341:bool)
                        n223 = case shown="True" w341 {
                          frame False {
                            n224 = property on="Laser Status" class="Bool (strict)"("Colors [4]"=cluster{u32, u32}[] [{16762130, 16762130}, {10441728, 10441728}, {10441728, 10441728}]) -> ()  [unwired: 2 in, 2 out]
                          }
                          frame True {
                            n225 = property on="Laser Status" class="Bool (strict)"("Colors [4]"=cluster{u32, u32}[] [{6618880, 6618880}]) -> ()  [unwired: 2 in, 2 out]
                          }
                        }
                      }
                      frame True {
                        w346 = FALSE
                        n226 = local write "Laser Control"(w346) -> ()
                        n227 = property on="Laser Status" class="Bool (strict)"("Colors [4]"=cluster{u32, u32}[] [{10682272, 10682272}, {12451729, 12451729}]) -> ()  [unwired: 2 in, 2 out]
                        "Laser Status" <- w346
                      }
                    }
                  }
                  frame True {
                    n228 = property on="Laser Status" class="Bool (strict)"("Colors [4]"=cluster{u32, u32}[] [{16723218, 15670016}, {16721170, 16725034}]) -> ()  [unwired: 2 in, 2 out]
                  }
                }
              }
              frame #3 {
                w351 = 2.0 ("y")
                w354 = 30
                n229 = Array Size(array=w349) -> (size(s)=w365:i32[])
                n230 = Index Array(array=w365, index=0) -> (element=w362:i32)
                n231 = Index Array(array=w365, index=1) -> (element=w361:i32)
                n232 = Multiply(x=w362, y=w361) -> (x*y=w359:i32)
                n233 = Divide(x=w359, y=w354) -> (x/y=w360:dbl)
                n234 = Divide(x=w354, y=w351) -> (x/y=w355:dbl)
                n235 = Reshape Array(w349, w359) -> (w358:string[])
                n236 = Subtract(x=w351, y=2.0) -> (x-y=w352:dbl)
                n237 = Round Toward +Infinity(x=w360) -> (ceil(x): smallest int >= x=w353:dbl)
                n238 = Initialize Array("", w355, w352) -> (w356:string[][])
                n239 = for {
                  N: w353 -> [_]
                  tunnel: w354 -> [w379]
                  shift-right: [w377] -> _
                  shift-left: w358 -> [w378]
                  tunnel: w354 -> [w373]
                  tunnel: w351 -> [w366]
                  shift-right: [w367] -> w348
                  shift-left: w356 -> [w369]
                  i -> [w376]
                  n240 = Divide(x=w373, y=w366) -> (x/y=w372:dbl)
                  n241 = Multiply(x=w376, y=w366) -> (x*y=w368:dbl)
                  n242 = Round Toward -Infinity(1:w372) -> (0:w371:dbl)
                  n243 = Split 1D Array(array=w378, index=w379) -> (first subarray=w375:string[], second subarray=w377:string[])
                  n244 = Reshape Array(w375, w371, 2 ("dimension size")) -> (w370:string[][])
                  n245 = Insert Into Array(array=w369, index (col)=w368, new element=w370) -> (w367:string[][])  [unwired: 1 in]
                }
                "Query List" <- w348
              }
              frame #4 {
                n246 = shared-variable ".\\Laser Library.lvlib\\Remote WV"() -> (w380:dbl)  [unwired: 1 in, 1 out]
                n247 = feedback-in #1(w380) -> ()
                n248 = feedback #1(w380) -> (w382:dbl)
                n249 = Not Equal?(x=w380, y=w382) -> (x != y?=w381:bool)
                n250 = case shown="True" w381 {
                  tunnel: w380 -> [_ w383]
                  frame False {
                  }
                  frame True {
                    n251 = property on="Wavelength" class="DigNum (strict)"("Val(Sgnl)"=w383) -> ()  [unwired: 2 in, 2 out]
                  }
                }
              }
            }
            n252 = local read "State next step"() -> (w266:string)
            "queue #" <- w265
          }
          frame "Walker" {
            w389 = dbl[] [680.0, 730.0, 780.0, 830.0, 880.0, 930.0, 980.0, 1030.0, 980.0, 930.0, 880.0, 830.0, 780.0, 730.0, 680.0, 800.0] ("Array")
            n253 = Wait (ms)(milliseconds to wait=2000) -> ()  [unwired: 1 out]
            n254 = local read "Step"() -> (w391:dbl)
            n255 = Index Array(array=w389, index=w391) -> (element=w385:dbl)
            n256 = Array Size(array=w389) -> (size(s)=w388:i32)
            n257 = Increment(x=w391) -> (x+1=w387:dbl)
            n258 = property on="Wavelength" class="DigNum (strict)"("Val(Sgnl)"=w385) -> ()  [unwired: 2 in, 2 out]
            n259 = Equal?(x=w387, y=w388) -> (x = y?=w386:bool)
            n260 = case shown="True" w386 {
              tunnel: w387 -> [w394 _]
              tunnel: [TRUE FALSE ("Walking")] -> w384
              frame False {
                n261 = local write "Step"(w394) -> ()
              }
              frame True {
                n262 = local write "WV Walk"(FALSE) -> ()
                n263 = local write "State next step"("Writer") -> ()
              }
            }
            "Walking" <- w384
          }
          frame "Backuper" {
            n264 = local read "Backuper state"() -> (w398:string)
            n265 = case shown="\"BackupInit\", Default" w398 {
              tunnel: w400 -> [_ w423]
              frame "BackupInit", Default {
                n266 = flat-sequence {
                  frame #0 {
                    n267 = Wait (ms)(milliseconds to wait=u32 30000) -> ()  [unwired: 1 out]
                    n268 = local write "Backuper state"("BackupFinal") -> ()
                  }
                  frame #1 {
                    n269 = local write "Refresh"(TRUE ("Refresh")) -> ()
                  }
                }
              }
              frame "BackupFinal" {
                n270 = local write "Backup"(FALSE ("Backup")) -> ()
                n271 = local write "State next step"("Writer") -> ()
                n272 = local write "Backuper state"("BackupInit") -> ()
                n273 = String To IP() -> (0:w416:u32)  [unwired: 1 in]
                n274 = IP To String(2:w416) -> (0:w404:string)  [unwired: 1 in]
                n275 = call "create unique folder.vi"("string"=w404, "path 2"=path "Y:/2PLaserBackup") -> ("path"=w409:path)  [unwired: 9 in]
                n276 = Get Date/Time In Seconds() -> (seconds since 1Jan1904=w419:timestamp)
                n277 = Format Date/Time String(time format string (%c)="%Y-%m-%d-%H-%M-%S", seconds (now)=w419) -> (date/time string=w413:string)  [unwired: 1 in]
                n278 = Path To String(path=w409) -> (string=w415:string)
                n279 = Concatenate Strings(w415, "\\" ("string"), w413, ".csv" ("string")) -> (w412:string)
                n280 = String To Path(string=w412) -> (path=w411:path)
                n281 = call-poly <vilib>:"Write To Spreadsheet File.vi"("delimiter (\\t)"="," ("delimiter (\\t)"), "format (%s)"="%.6f" ("format (%.3f)"), "append to file? (new file:F)"=FALSE, "2D data"=w423, "file path (dialog if empty)"=w411) -> ()  [unwired: 2 in, 2 out]
                "Backing up" <- FALSE ("Backing up ...")
              }
            }
          }
          frame "Quiter" {
            n282 = Equal To 0?(x=w427) -> (x = 0?=w426:bool)
            n283 = case shown="False" w426 {
              tunnel: ["Quiter" "Writer"] -> w425
              tunnel: [_ w430] -> w424
              frame False {
              }
              frame True {
                n284 = local read "Sleep"() -> (w429:bool)
                n285 = case shown="True" w429 {
                  tunnel: [w432 _] -> w430
                  frame False {
                    w432 = TRUE
                    n286 = local write "QUIT"(FALSE) -> ()
                    n287 = local write "stop"(w432) -> ()
                  }
                  frame True {
                    n288 = local write "Sleep"(FALSE ("Sleep")) -> ()
                    n289 = local write "State next step"("Writer" ("State next step")) -> ()
                  }
                }
              }
            }
          }
        }
      }
      n290 = VISA Close(VISA resource name=w47, error in (no error)=w46) -> (error out=w52:errorcluster)
      n291 = call <vilib>:"Simple Error Handler.vi"("error in (no error)"=w52) -> ()  [unwired: 1 in, 8 out]
    }
  }
